vi "read data 1  (SubVI).vi"() -> (2 "read data":u8 format="%x", 3 "data's booleans":bool[](array[boolean]))   [LabVIEW 2019]
uses:
  <vilib>/rvi/eio/common/nirviEmuTemplateMethod_errors.vi
  <vilib>/eio/EIONode/EIONode.xnode
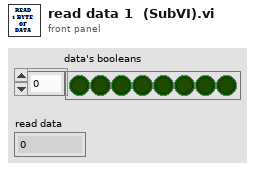
[diagram p1: front panel]
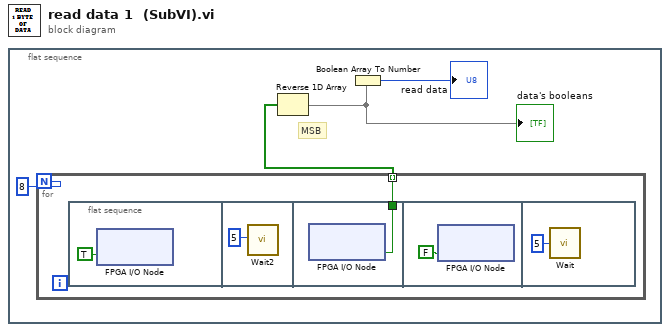
[diagram p0: block diagram]
diagram:
  n1 = flat-sequence {
    frame #0 {
      # "MSB"
      n2 = for {
        N: 8 -> [_]
        tunnel: [w5] -> w3 mode=indexing
        n3 = flat-sequence {
          tunnel: [w8] -> w5
          frame #0 {
            n4 = xnode "FPGA I/O Node"("SCL"=TRUE) -> ()  [unwired: 1 in, 1 out]
          }
          frame #1 {
            n5 = call "Wait2"("Count(uSec)"=u32 5 ("Count(Ticks)")) -> ()  [unwired: 1 out]
          }
          frame #2 {
            n6 = xnode "FPGA I/O Node"() -> ("SDA"=w8:bool)  [unwired: 1 in, 1 out]
          }
          frame #3 {
            n7 = xnode "FPGA I/O Node"("SCL"=FALSE) -> ()  [unwired: 1 in, 1 out]
          }
          frame #4 {
            n8 = call "Wait"("Count(uSec)"=u32 5 ("Count(Ticks)")) -> ()  [unwired: 1 out]
          }
        }
      }
      n9 = Reverse 1D Array(array=w3) -> (reversed array=w1:bool[])
      "data's booleans" <- w1
      n10 = Boolean Array To Number(Boolean array=w1) -> (number=→"read data":u8)
    }
  }
